vi "getOffsetToUTC.vi"(11 "Epoch (UNIX)":refnum<class "Epoch.UNIX.lvclass">) -> (2 "Offset to UTC":i64)   [LabVIEW 2013, in "Epoch.UNIX.lvclass"]
uses:
  Epoch.UNIX.lvclass
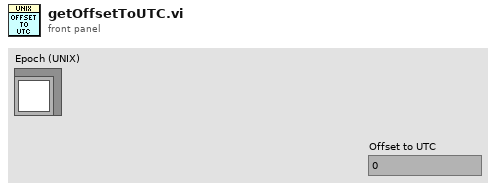
[diagram p1: front panel]
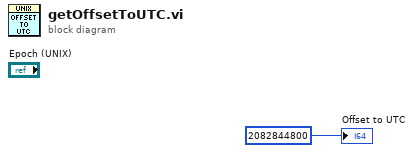
[diagram p0: block diagram]
diagram:
  "Offset to UTC" <- i64 2082844800 ("Timestamp Offset")
